vi "Read Element of Tree.vi"(8 "error in (no error)":errorcluster, 10 "index":i32, 11 "Fast Tree in":refnum<class "Fast Tree.lvclass">) -> (0 "error out":errorcluster, 2 "Node":T1={"Record Type"="", "Payload"="", "Parent Index"=-1, "First Child Index"=-1, "Next Sibling Index"=-1}, 3 "Fast Tree out":refnum<class "Fast Tree.lvclass">)   [LabVIEW 2019, in "Fast Tree.lvclass"]
uses:
  Fast Tree.lvclass
  Fast Tree.lvclass/Fast Tree.ctl
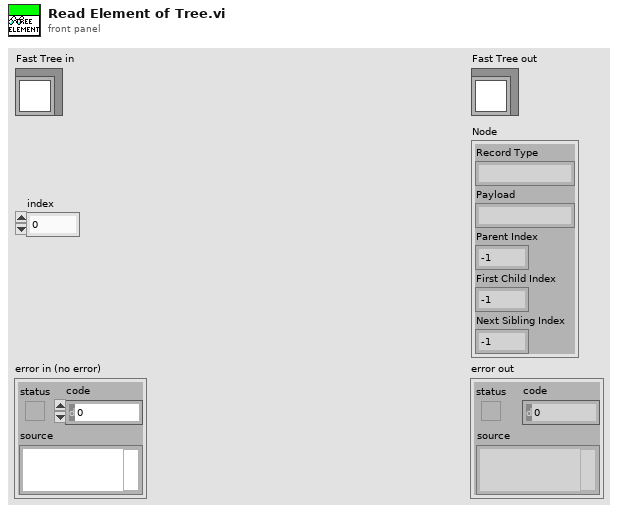
[diagram p1: front panel]
types:
  T1 = cluster{"Record Type":string, "Payload":string, "Parent Index":i32, "First Child Index":i32, "Next Sibling Index":i32}
  T2 = cluster{"Record Type":string, "Payload":string, "Parent Index":i32, "First Child Index":i32, "Next Sibling Index":i32}[]
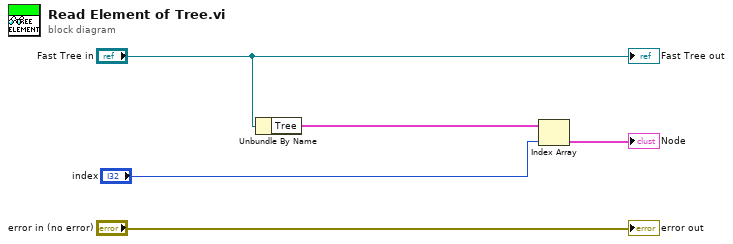
[diagram p0: block diagram]
diagram:
  n1 = Unbundle By Name("Fast Tree in") -> ("Tree"=w2:T2)
  n2 = Index Array(array=w2, index="index") -> (element=→"Node":T1)
  "error out" <- "error in (no error)"
  "Fast Tree out" <- "Fast Tree in"
